vi "receiveMessage.vi"(0 "connection ID":refnum<k5>, 1 "error in":errorcluster) -> (2 "data out":string, 3 "connection ID out":refnum<k5>, 4 "error out":errorcluster)   [LabVIEW 2023]
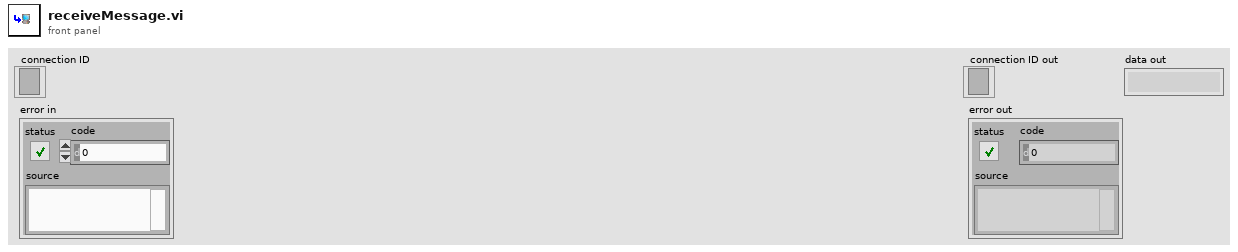
[diagram p1: front panel]
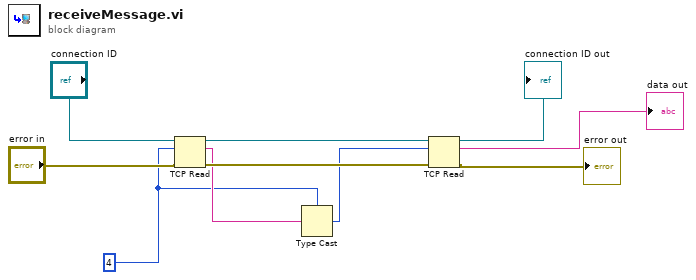
[diagram p0: block diagram]
diagram:
  w3 = 4
  n1 = TCP Read(connection ID="connection ID", bytes to read=w3, error in (no error)="error in") -> (connection ID out=w9:refnum<k5>, data out=w4:string, error out=w10:errorcluster)  [unwired: 2 in]
  n2 = Type Cast(type=w3, x=w4) -> (*(type *) &x=w2:i32)
  n3 = TCP Read(connection ID=w9, bytes to read=w2, error in (no error)=w10) -> (connection ID out=→"connection ID out":refnum<k5>, data out=→"data out":string, error out=→"error out":errorcluster)  [unwired: 2 in]
